vi "FTW-Test-JSON-Deserialize.vi"() -> (0 "Test Result":errorcluster)   [LabVIEW 2014]
uses:
  lib/FTW-LibraryFilepath.vi
  src/core/reflection/FTW-Reflection-Type.vi
  src/core/error/FTW-ERR-ThrowGenericError.vi
  src/core/error/FTW-ERR-Assert-DeveloperError.vi
  src/core/error/FTW-ERR-ThrowError.vi
  src/core/error/FTW-ERR-CallChain.vi
  src/core/string/FTW-STR-ReplaceWhitespace.vi
  src/core/reflection/FTW-Reflection-Array.vi
  src/core/json/core/FTW-JSON-Core-GetFlattenedValue.vi
  src/core/json/FTW-JSON-Deserialize/FTW-JSON-Deserialize.xnode
panel:
  out "JSON String (UTF-8)":string
  out "Array":i64[](array[numeric])
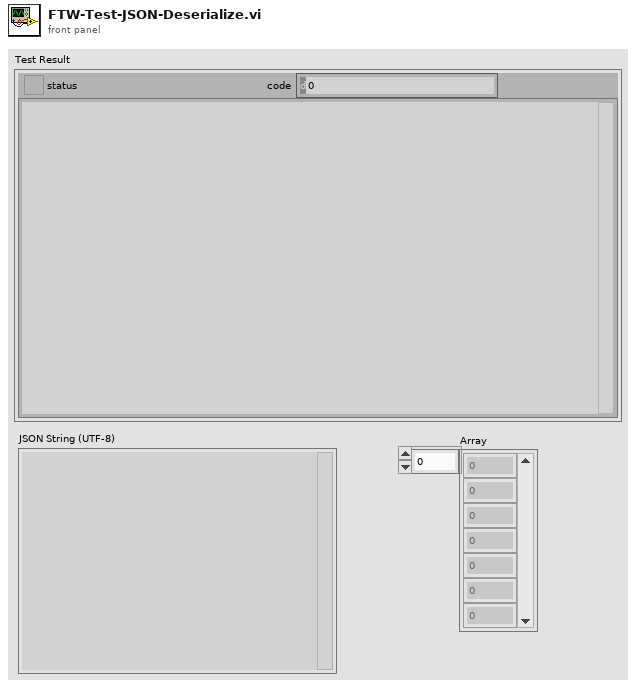
[diagram p1: front panel]
types:
  T1 = cluster{"LoggerAddress":string, "BooleanTrue":bool}
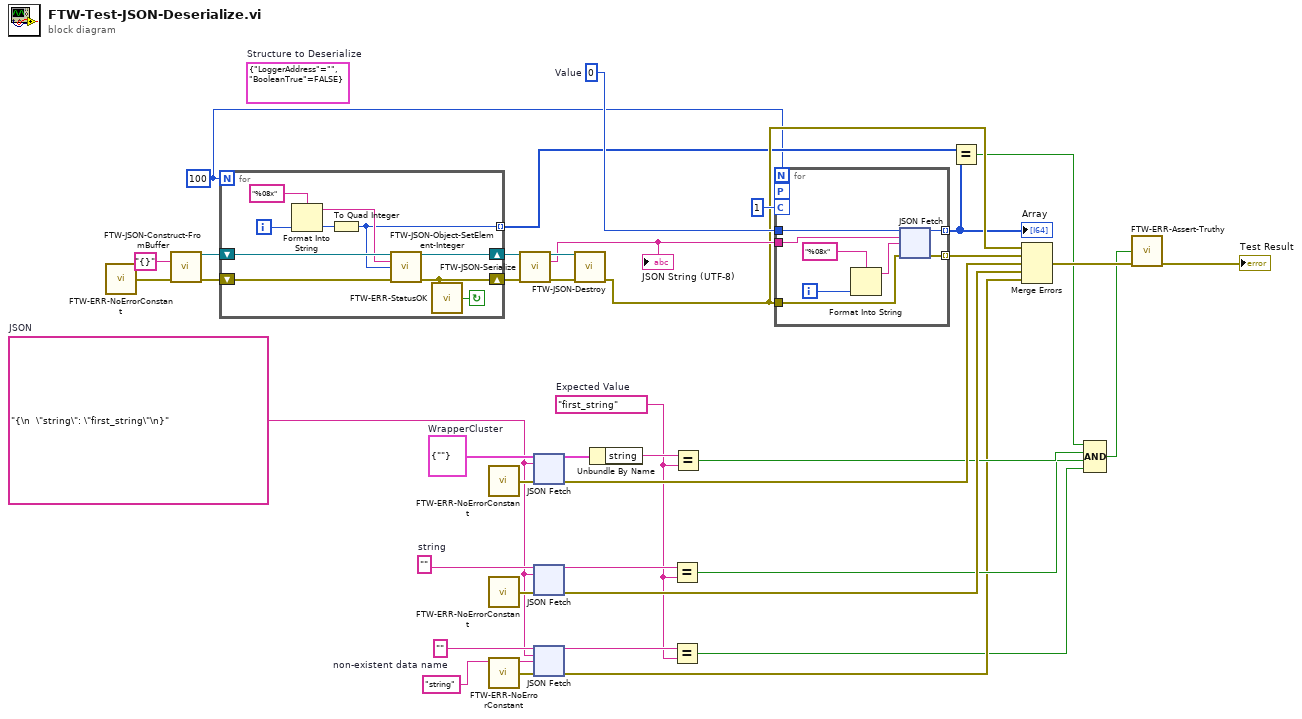
[diagram p0: block diagram]
diagram:
  w2 = ""  # non-existent data name
  w19 = ""  # string
  w5 = "first_string"  # Expected Value
  w1 = "{\n  \"string\": \"first_string\"\n}"  # JSON
  w21 = cluster{"string":string} {"string"=""}  # WrapperCluster
  w29 = i64 0  # Value
  w22 = 100
  (unwired) T1 {"LoggerAddress"="", "BooleanTrue"=FALSE}  # Structure to Deserialize
  n1 = call "FTW-ERR-NoErrorConstant.vi"() -> ("no error"=w37:errorcluster)
  n2 = call "FTW-JSON-Construct-FromBuffer.vi"("JSON String (UTF-8)"="{}", "error in"=w37) -> ("JSON Object"=w33:refnum<data-value>, "error out"=w32:errorcluster)  [unwired: 12 in]
  n3 = for {
    N: w22 -> [_]
    shift-right: [w42] -> w35
    shift-left: w32 -> [w46]
    shift-right: [w47] -> w36
    shift-left: w33 -> [w48]
    tunnel: [w40] -> w25 mode=indexing
    i -> [w45]
    stop <- w41 continue-if-true
    n4 = Format Into String(format string="%08x", w45) -> (resulting string=w44:string)  [unwired: 2 in, 1 out]
    n5 = To Quad Integer(1:w45) -> (0:w40:i64)
    n6 = call "FTW-JSON-Object-SetElement-Integer.vi"("JSON Object"=w48, "Key"=w44, "Value"=w40, "error in"=w46) -> ("JSON Object out"=w47:refnum<data-value>, "error out"=w42:errorcluster)  [unwired: 10 in]
    n7 = call "FTW-ERR-StatusOK.vi"("error to check"=w42) -> ("Status OK?"=w41:bool)
  }
  n8 = call "FTW-ERR-NoErrorConstant.vi"() -> ("no error"=w18:errorcluster)
  n9 = call "FTW-ERR-NoErrorConstant.vi"() -> ("no error"=w17:errorcluster)
  n10 = call "FTW-ERR-NoErrorConstant.vi"() -> ("no error"=w8:errorcluster)
  n11 = call "FTW-JSON-Serialize.vi"("JSON Object"=w36, "error in"=w35) -> ("JSON Object out"=w34:refnum<data-value>, "JSON String (UTF-8)"=w30:string, "error out"=w31:errorcluster)  [unwired: 11 in]
  "JSON String (UTF-8)" <- w30
  n12 = xnode "JSON Fetch"("Type and Defaults"=w21, "JSON String"=w1, "error in"=w18) -> ("Values"=w20:cluster{"string":string}, "error out"=w14:errorcluster)  [unwired: 1 in]
  n13 = xnode "JSON Fetch"("Type and Defaults"=w19, "JSON String"=w1, "error in"=w17) -> ("Values"=w15:string, "error out"=w13:errorcluster)  [unwired: 1 in]
  n14 = xnode "JSON Fetch"("Type and Defaults"=w2, "JSON String"=w1, "Element Path"="string", "error in"=w8) -> ("Values"=w6:string, "error out"=w4:errorcluster)
  n15 = call "FTW-JSON-Destroy.vi"("JSON Object"=w34, "error in"=w31) -> ("error out"=w27:errorcluster)  [unwired: 13 in]
  n16 = Unbundle By Name(w20) -> ("string"=w16:string)
  n17 = Equal?(x=w15, y=w5) -> (x = y?=w9:bool)
  n18 = Equal?(x=w6, y=w5) -> (x = y?=w3:bool)
  n19 = Equal?(x=w16, y=w5) -> (x = y?=w10:bool)
  n20 = for {
    N: w22 -> [_]
    workers-P: _ -> [_]
    tunnel: w29 -> [w56]
    chunk-C: 1 -> [_]
    tunnel: w30 -> [w55]
    tunnel: [w51] -> w26 mode=indexing
    tunnel: [w50] -> w28 mode=indexing
    tunnel: w27 -> [w49]
    i -> [w53]
    n21 = Format Into String(format string="%08x", w53) -> (resulting string=w54:string)  [unwired: 2 in, 1 out]
    n22 = xnode "JSON Fetch"("Type and Defaults"=w56, "JSON String"=w55, "Element Path"=w54, "error in"=w49) -> ("Values"=w51:i64, "error out"=w50:errorcluster)
  }
  "Array" <- w26
  n23 = Equal?(x=w25, y=w26) -> (x = y?=w12:bool)
  n24 = Merge Errors(w27, w28, w14, w13, w4) -> (w24:errorcluster)
  n25 = Compound Arithmetic op=AND(w12, w10, w9, w3) -> (w11:bool)
  n26 = call "FTW-ERR-Assert-Truthy.vi"("Expected Truthy"=w11, "error in"=w24) -> ("error out"=→"Test Result":errorcluster)  [unwired: 13 in]
